vi "Calculate Thermistor Temp.vi"(11 "Input":dbl=2.421875) -> (3 "Output":dbl=24.490923291015623)   [LabVIEW 2015]
panel:
  in  "C":dbl=-17.6124
  in  "B":dbl=11.1259
  in  "A":dbl=2.3306
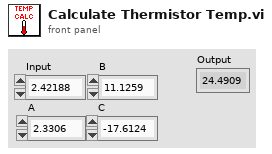
[diagram p1: front panel]
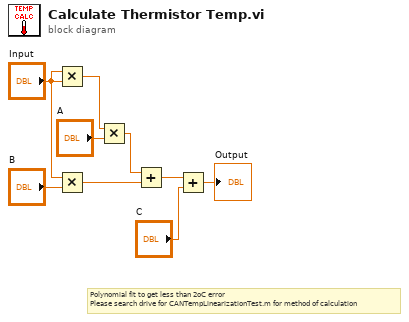
[diagram p0: block diagram]
diagram:
  # "Polynomial fit to get less than 2oC error\nPlease search drive for CANTempLinearizationTest.m for method of calculation"
  n1 = Multiply(x="Input", y="Input") -> (x*y=w8:dbl)
  n2 = Multiply(x="Input", y="B") -> (x*y=w6:dbl)
  n3 = Multiply(x=w8, y="A") -> (x*y=w7:dbl)
  n4 = Add(x=w7, y=w6) -> (x+y=w5:dbl)
  n5 = Add(x=w5, y="C") -> (x+y=→"Output":dbl)
